vi "TestExec.Test ID - Update Test SectionX.vi"(10 "TC Cnts":i32[](array[numeric]), 11 "Start(T)/End(F)":bool) -> (0 "Test ID":string, 1 "TC Level Out":i32, 2 "TC Cnts Out":i32[](array[numeric]))   [LabVIEW 2016]
panel:
  out "TC Level Out 2":i32
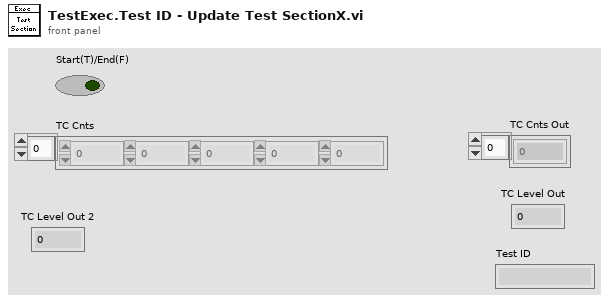
[diagram p1: front panel]
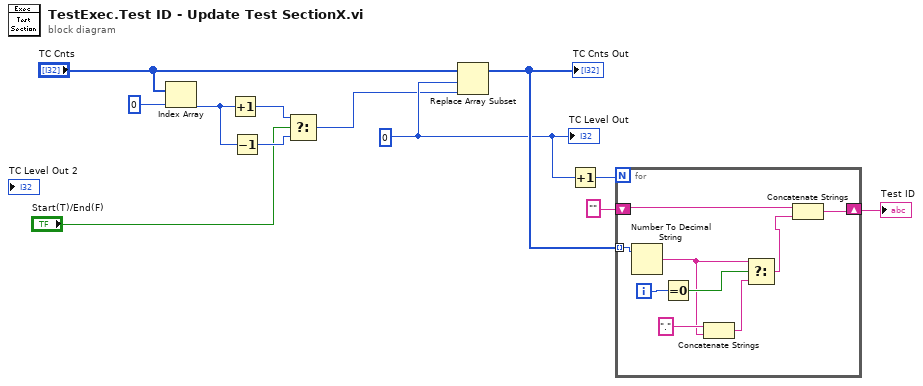
[diagram p0: block diagram]
diagram:
  w9 = 0
  n1 = Index Array(array="TC Cnts", index=0) -> (element=w5:i32)
  n2 = Increment(x=w5) -> (x+1=w4:i32)
  n3 = Decrement(x=w5) -> (x-1=w3:i32)
  n4 = Select(t=w4, s="Start(T)/End(F)", f=w3) -> (s? t:f=w1:i32)
  n5 = Replace Array Subset(array="TC Cnts", new element=w1, index=w9) -> (w11:i32[])
  "TC Cnts Out" <- w11
  n6 = Increment(x=w9) -> (x+1=w10:i32)
  n7 = for {
    N: w10 -> [_]
    tunnel: w11 -> [w20] mode=indexing
    shift-right: [w15] -> w7
    shift-left: "" -> [w14]
    i -> [w21]
    n8 = Number To Decimal String(number=w20) -> (decimal integer string=w16:string)  [unwired: 1 in]
    n9 = Equal To 0?(x=w21) -> (x = 0?=w17:bool)
    n10 = Concatenate Strings(".", w16) -> (w18:string)
    n11 = Select(t=w16, s=w17, f=w18) -> (s? t:f=w13:string)
    n12 = Concatenate Strings(w14, w13) -> (w15:string)
  }
  "Test ID" <- w7
  "TC Level Out" <- w9
